vi "Read_Alicat_Diff.vi"(10 "Device ID":string, 11 "VISA Sesssion In":refnum<visa-resource-name>="ASRL13::INSTR") -> (0 "error out":errorcluster, 2 "Pressure Out":string, 3 "VISA Sesssion Out":refnum<visa-resource-name>="ASRL6::INSTR")   [LabVIEW 2019]
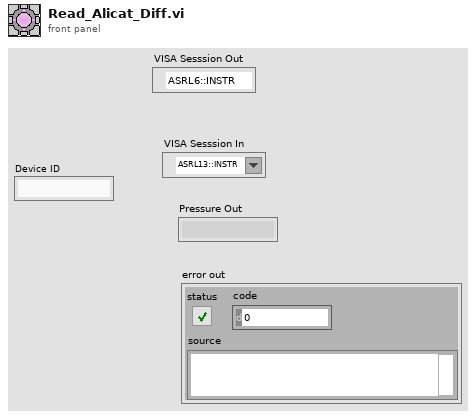
[diagram p1: front panel]
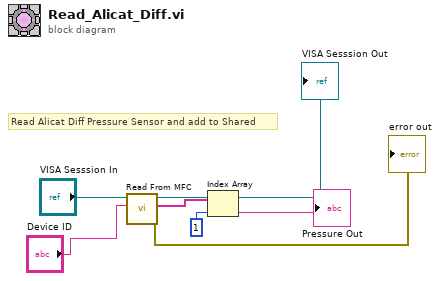
[diagram p0: block diagram]
diagram:
  # "Read Alicat Diff Pressure Sensor and add to Shared"
  n1 = call "Read From MFC.vi"("Device ID"="Device ID", "VISA Sesssion In"="VISA Sesssion In") -> ("error out"=→"error out":errorcluster, "Output"=w7:string[], "VISA Sesssion Out"=→"VISA Sesssion Out":refnum<visa-resource-name>)  [unwired: 7 in]
  n2 = Index Array(array=w7, index=1) -> (element=→"Pressure Out":string)
